vi "Read Msg Update.vi"(8 "error in (no error)":errorcluster, 11 "Connection Listener in":refnum<class "Connection Listener.lvclass">) -> (0 "error out":errorcluster, 2 "Msg Update":refnum<user-event>, 3 "Connection Listener out":refnum<class "Connection Listener.lvclass">)   [LabVIEW 2017, in "Connection Listener.lvlib" / "Connection Listener.lvclass"]
uses:
  Connection Listener.lvclass
  Connection Listener.lvclass/Connection Listener.ctl
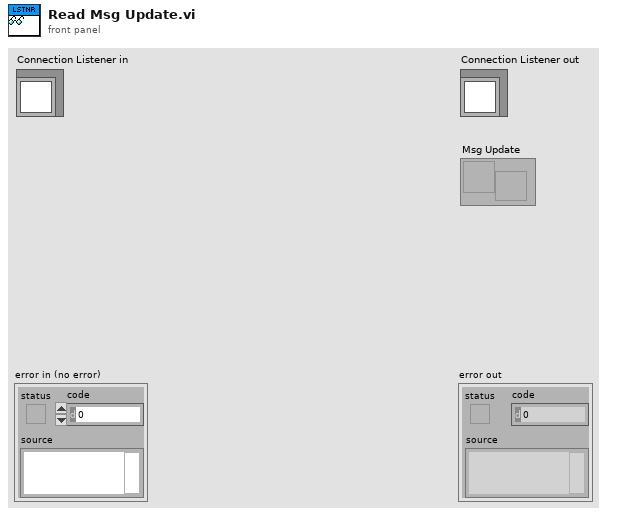
[diagram p1: front panel]
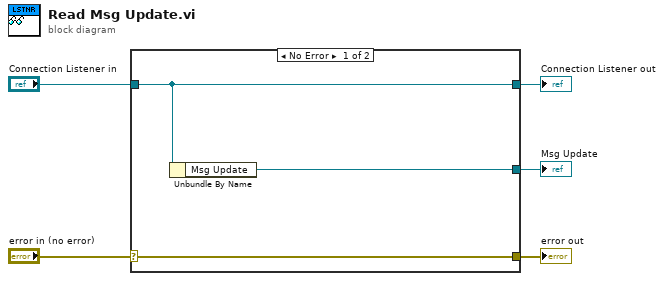
[diagram p0: block diagram]
diagram:
  n1 = case shown="No Error" "error in (no error)" {
    selector: "error in (no error)" -> [w8 w9]
    tunnel: [w8 w9] -> w4
    tunnel: [w7 w10] -> w2
    tunnel: "Connection Listener in" -> [w7 w10]
    tunnel: [w6 _] -> w1
    frame No Error {
      n2 = Unbundle By Name(w7) -> ("Msg Update"=w6:refnum<user-event>)
    }
    frame Error {
    }
  }
  "error out" <- w4
  "Connection Listener out" <- w2
  "Msg Update" <- w1
